vi "Warn.vi"(8 "error in (no error)":errorcluster, 11 "Message":string) -> (0 "error out":errorcluster)   [LabVIEW 2016, in "Log4Lv.lvlib"]
doc: "Use this template to build a VI to use as a subVI."
uses:
  Log4Lv.lvlib
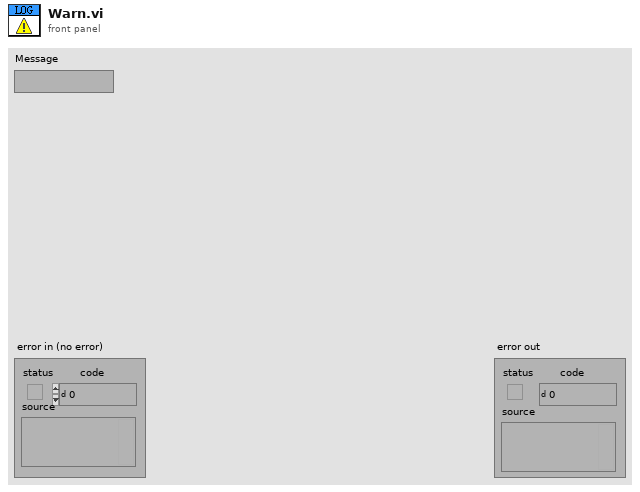
[diagram p1: front panel]
types:
  T1 = enum16{"Disable", "Error", "Warn", "Info", "Debug"}
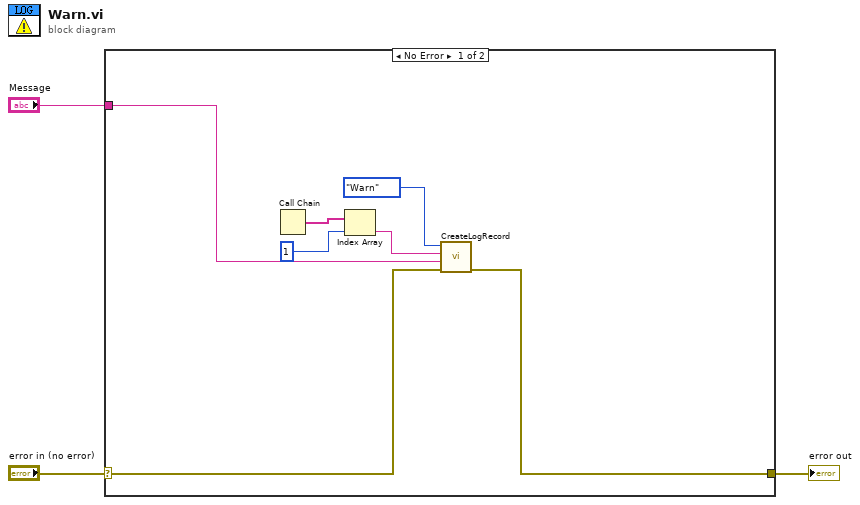
[diagram p0: block diagram]
diagram:
  n1 = case shown="No Error" "error in (no error)" {
    selector: "error in (no error)" -> [w6 w11]
    tunnel: [w5 w11] -> w2
    tunnel: "Message" -> [w4 _]
    frame No Error {
      n2 = Call Chain() -> (call chain=w9:string[])
      n3 = Index Array(array=w9, index=1) -> (element=w8:string)
      n4 = call "CreateLogRecord.vi"("error in (no error)"=w6, "Message"=w4, "Source"=w8, "Level"=T1."Warn") -> ("error out"=w5:errorcluster)  [unwired: 7 in]
    }
    frame Error {
    }
  }
  "error out" <- w2
